vi "VI-Find Wire.vi"(0 "VI in":refnum<vi>, 7 "Terms":string[](array[string]), 11 "error in (no error)":errorcluster) -> (4 "VI out":refnum<vi>, 8 "Wire Refnum":refnum<vi>, 15 "error out":errorcluster)   [LabVIEW 2015]
uses:
  <vilib>/Utility/traverseref.llb/TRef TravTarget.ctl
  <vilib>/Utility/traverseref.llb/VI Scripting - Traverse.lvlib
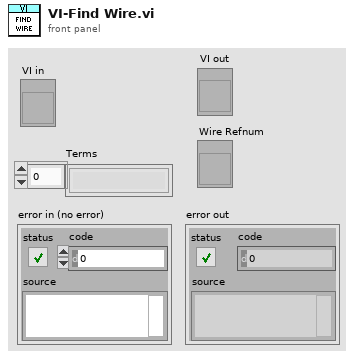
[diagram p1: front panel]
types:
  T1 = typedef "TRef TravTarget.ctl" = enum16{"FP", "BD", "Other"}
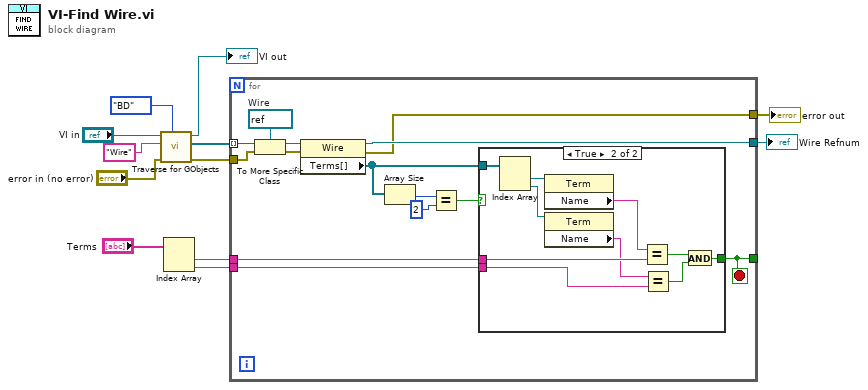
[diagram p0: block diagram]
diagram:
  n1 = call <vilib>:"Traverse for GObjects.vi"("Traverse Target"=TRef_TravTarget."BD", "error in (no error)"="error in (no error)", "Class Name"="Wire", "VI Refnum"="VI in") -> ("error out"=w2:errorcluster, "References"=w12:refnum<vi>[], "dup VI Refnum"=→"VI out":refnum<vi>)  [unwired: 4 in, 1 out]
  n2 = Index Array(array="Terms") -> (element #1=w5:string, element #2=w4:string)  [unwired: 2 in]
  n3 = for {
    tunnel: w12 -> [w25] mode=indexing
    tunnel: [w19] -> w3
    tunnel: w5 -> [w18]
    tunnel: w4 -> [w17]
    tunnel: [w16] -> _
    tunnel: w2 -> [w15]
    tunnel: [w13] -> w1
    stop <- w16 stop-if-true
    w26 = refnum<vi> refnum  # Wire
    n4 = To More Specific Class(target class=w26, reference=w25, error in=w15) -> (specific class reference=w24:refnum<vi>, error out=w14:errorcluster)
    n5 = property class="Wire"(reference=w24, error in=w14) -> (reference out=w19:refnum<vi>, error out=w13:errorcluster, "Terms[]"=w20:refnum<vi>[])
    n6 = Array Size(array=w20) -> (size(s)=w23:i32)
    n7 = Equal?(x=w23, y=2) -> (x = y?=w21:bool)
    n8 = case shown="True" w21 {
      tunnel: w20 -> [_ w36]
      tunnel: w18 -> [_ w32]
      tunnel: w17 -> [_ w30]
      tunnel: [_ w27] -> w16
      frame False {
      }
      frame True {
        n9 = Index Array(array=w36) -> (element #1=w35:refnum<vi>, element #2=w34:refnum<vi>)  [unwired: 2 in]
        n10 = property class="Term"(reference=w35) -> ("Name"=w33:string)  [unwired: 1 in, 2 out]
        n11 = property class="Term"(reference=w34) -> ("Name"=w31:string)  [unwired: 1 in, 2 out]
        n12 = Equal?(x=w33, y=w32) -> (x = y?=w29:bool)
        n13 = Equal?(x=w31, y=w30) -> (x = y?=w28:bool)
        n14 = And(x=w29, y=w28) -> (x .and. y?=w27:bool)
      }
    }
  }
  "error out" <- w1
  "Wire Refnum" <- w3
